vi "Get Error.vi"(8 "error in (no error)":errorcluster, 11 "DOM document in":refnum<k20>) -> (0 "error out":errorcluster, 2 "errors":T1[](array[typedef]), 3 "DOM document out":refnum<k20>)   [LabVIEW 2017, in "Error File Management.lvlib"]
uses:
  Error File Management.lvlib
  Controls/NI Error.ctl
  <vilib>/xml/Close Reference(Node).vi
  <vilib>/xml/NI_XML.lvlib
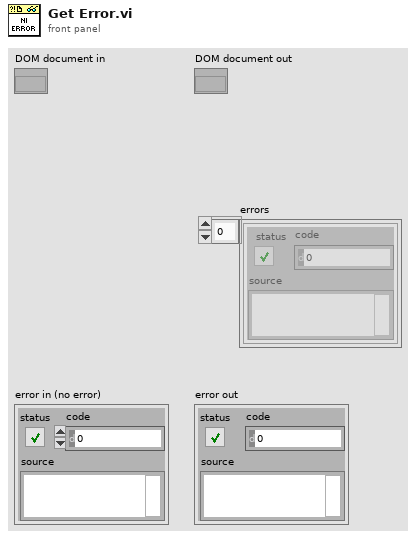
[diagram p1: front panel]
types:
  T1 = typedef "Error File Management.lvlib/NI Error.ctl" = errorcluster
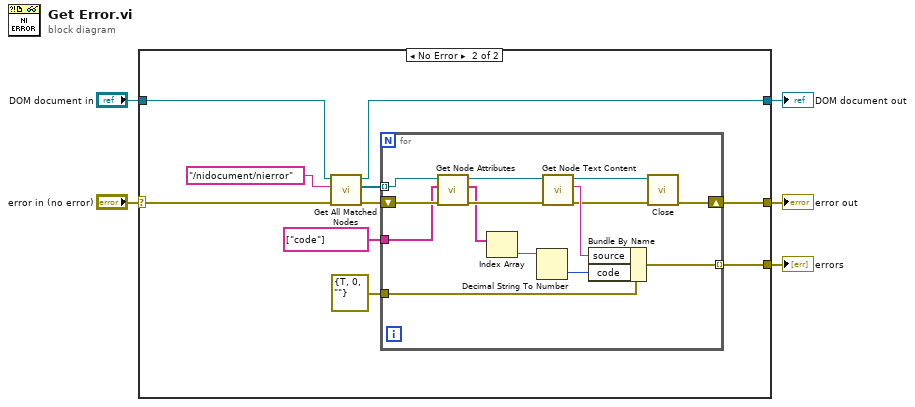
[diagram p0: block diagram]
diagram:
  n1 = case shown="No Error" "error in (no error)" {
    selector: "error in (no error)" -> [w7 w9]
    tunnel: [_ w17] -> w1
    tunnel: [w6 w13] -> w5
    tunnel: "DOM document in" -> [w6 w12]
    tunnel: [w7 w10] -> w2
    frame Error {
    }
    frame No Error {
      n2 = call <vilib>:"Get All Matched Nodes.vi"("error in (no error)"=w9, "XPath expression"="/nidocument/nierror", "node in"=w12) -> ("error out"=w16:errorcluster, "node result array"=w15:refnum<k20>[], "node out"=w13:refnum<k20>)  [unwired: 6 in]
      n3 = for {
        tunnel: w15 -> [w28] mode=indexing
        shift-right: [w31] -> w10
        shift-left: w16 -> [w27]
        tunnel: [w30] -> w17 mode=indexing
        tunnel: string[] ["code"] -> [w26]
        tunnel: T1 {"status"=TRUE, "code"=0, "source"=""} ("error") -> [w19]
        n4 = call "Get Node Attributes.vi"("error in (no error)"=w27, "names"=w26, "node in"=w28) -> ("error out"=w25:errorcluster, "values"=w23:string[], "node out"=w24:refnum<k20>)  [unwired: 6 in]
        n5 = Index Array(array=w23) -> (element=w22:string)  [unwired: 1 in]
        n6 = Decimal String To Number(string=w22) -> (number=w20:i32)  [unwired: 2 in, 1 out]
        n7 = call "Get Node Text Content.vi"("error in (no error)"=w25, "node in"=w24) -> ("error out"=w18:errorcluster, "node text"=w21:string, "node out"=w29:refnum<k20>)  [unwired: 7 in]
        n8 = Bundle By Name(cluster=w19, "source"=w21, "code"=w20) -> (w30:T1)
        n9 = call-poly <vilib>:"Close.vi"("error in (no error)"=w18, "node"=w29) -> ("error out"=w31:errorcluster)  [unwired: 7 out]
      }
    }
  }
  "DOM document out" <- w5
  "error out" <- w2
  "errors" <- w1
